vi "Keysight E36300 Series Output DC Volts.vi"(6 "Simulate":bool, 8 "Current Level (2 A)":dbl=2.0, 9 "Voltage Level (1 V)":dbl=1.0, 10 "Channel (1)":string="1", 11 "VISA resource name":refnum<visa-resource-name>) -> ()   [LabVIEW 2020]
doc: "This example shows how to configure the output DC volts."
uses:
  Keysight E36300 Series.lvlib
panel:
  out "Actual Voltage Level (V)":dbl[](array[numeric]) format="%.3g"
  out "Actual Current Level (A)":dbl[](array[numeric]) format="%.3g"
  # "(c) 2019 - 2021 National Instruments.  ALL RIGHTS RESERVED."
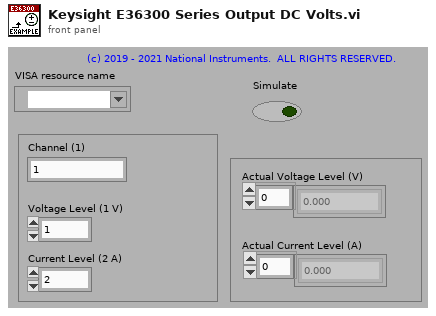
[diagram p1: front panel]
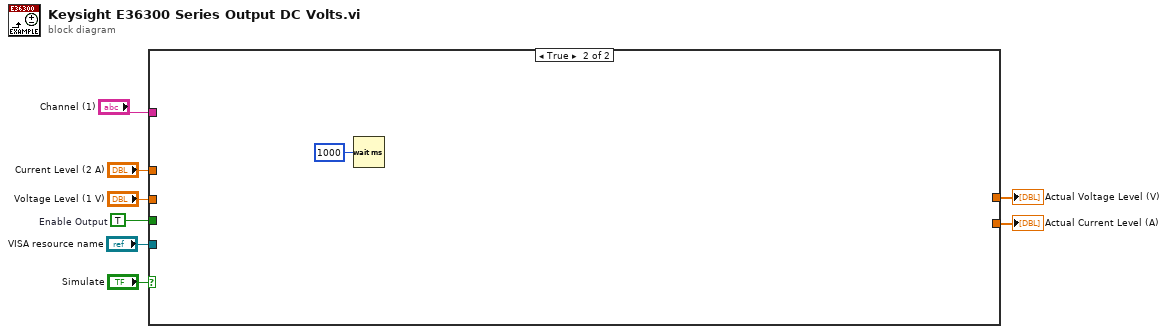
[diagram p0: block diagram]
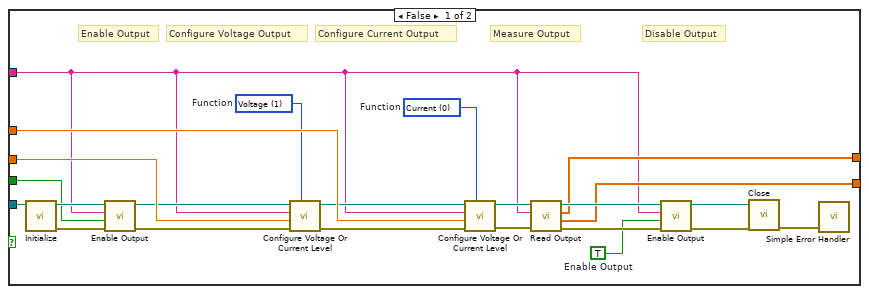
[diagram p2: hidden frame]
diagram:
  w6 = TRUE  # Enable Output
  n1 = case shown="True" "Simulate" {
    tunnel: "VISA resource name" -> [w31 _]
    tunnel: "Voltage Level (1 V)" -> [w29 _]
    tunnel: w6 -> [w21 _]
    tunnel: [w18 _] -> w5
    tunnel: [w17 _] -> w4
    tunnel: "Current Level (2 A)" -> [w15 _]
    tunnel: "Channel (1)" -> [w9 _]
    frame False {
      w13 = 0 items=["Current", "Voltage"]  # Function
      w14 = 1 items=["Current", "Voltage"]  # Function
      w20 = TRUE  # Enable Output
      # "Disable Output"
      # "Configure Current Output"
      # "Configure Voltage Output"
      # "Measure Output"
      # "Enable Output"
      n2 = call "Initialize.vi"("VISA resource name"=w31) -> ("error out"=w27:errorcluster, "VISA resource name out"=w28:refnum<visa-resource-name>)  [unwired: 9 in]
      n3 = call "Enable Output.vi"("error in (no error)"=w27, "Enable Output (F: Disable)"=w21, "Channel (1)"=w9, "VISA resource name"=w28) -> ("error out"=w19:errorcluster, "VISA resource name out"=w26:refnum<visa-resource-name>)  [unwired: 6 in]
      n4 = call "Configure Voltage Or Current Level.vi"("Function (0 : Current)"=w14, "error in (no error)"=w19, "Voltage Or Current Level (1)"=w29, "Channel (1)"=w9, "VISA resource name"=w26) -> ("error out"=w11:errorcluster, "VISA resource name out"=w10:refnum<visa-resource-name>)  [unwired: 5 in]
      n5 = call "Configure Voltage Or Current Level.vi"("Function (0 : Current)"=w13, "error in (no error)"=w11, "Voltage Or Current Level (1)"=w15, "Channel (1)"=w9, "VISA resource name"=w10) -> ("error out"=w12:errorcluster, "VISA resource name out"=w16:refnum<visa-resource-name>)  [unwired: 5 in]
      n6 = call "Read Output.vi"("error in (no error)"=w12, "Channel (1)"=w9, "VISA resource name"=w16) -> ("error out"=w23:errorcluster, "Actual Current Level (A)"=w17:dbl[], "Actual Voltage Level (V)"=w18:dbl[], "VISA resource name out"=w25:refnum<visa-resource-name>)  [unwired: 5 in]
      n7 = call "Enable Output.vi"("error in (no error)"=w23, "Enable Output (F: Disable)"=w20, "Channel (1)"=w9, "VISA resource name"=w25) -> ("error out"=w22:errorcluster, "VISA resource name out"=w24:refnum<visa-resource-name>)  [unwired: 6 in]
      n8 = call "Close.vi"("error in (no error)"=w22, "VISA resource name"=w24) -> ("error out"=w30:errorcluster)  [unwired: 9 in]
      n9 = call <vilib>:"Simple Error Handler.vi"("error in (no error)"=w30) -> ()  [unwired: 4 in, 5 out]
    }
    frame True {
      n10 = Wait (ms)(milliseconds to wait=u32 1000) -> ()  [unwired: 1 out]
    }
  }
  "Actual Current Level (A)" <- w4
  "Actual Voltage Level (V)" <- w5
